vi "LLTF_Contrast_Demo_Advanced.vi"() -> ()   [LabVIEW 2017]
uses:
  PE_Filter_SDK/PE_Filter_SDK.lvlib
panel:
  out "Grating Name":string
  in  "Grating":i32=4 min=0 max=2 step=1
  in  "Wavelength":dbl=600.0 min=500.0 max=600.0 format="%.2f"
  out "Min Ext. Wavelength":dbl
  out "Max Ext. Wavelength":dbl
  in  "Move Filter":bool
  in  "Stop":bool
  out "Grating Count":i32
  out "Current System":string
  in  "Configuration File":path
  # "Filter Selection"
  # "Filter Information"
  # "Filter Control"
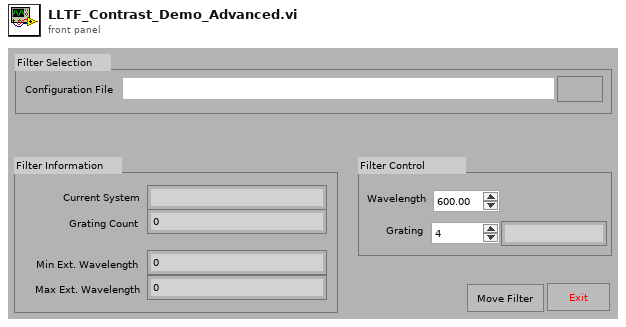
[diagram p1: front panel]
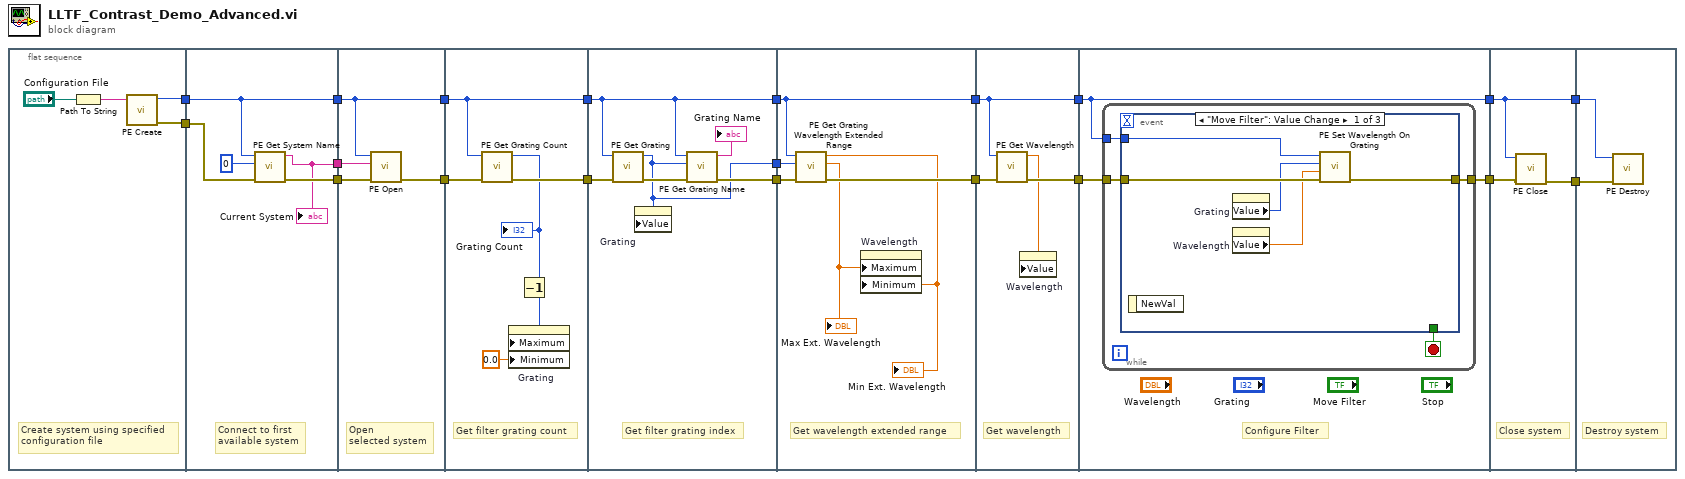
[diagram p0: block diagram]
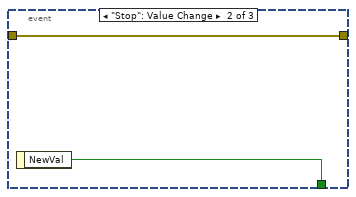
[diagram p2: hidden frame]
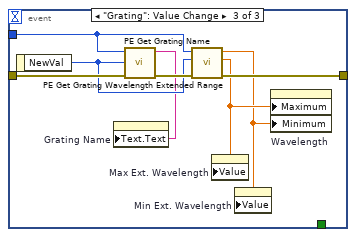
[diagram p3: hidden frame]
diagram:
  n1 = flat-sequence {
    tunnel: [w21] -> w20
    tunnel: [w22] -> w19
    tunnel: w20 -> [w29]
    tunnel: [w27] -> w17
    tunnel: [w28] -> w18
    tunnel: w19 -> [w26]
    tunnel: [w26] -> w16
    tunnel: w18 -> [w33]
    tunnel: [w30] -> w15
    tunnel: w17 -> [w32]
    tunnel: w16 -> [w31]
    tunnel: [w31] -> w14
    tunnel: w15 -> [w37]
    tunnel: [w38] -> w9
    tunnel: w14 -> [w39]
    tunnel: [w39] -> w8
    tunnel: w9 -> [w45]
    tunnel: [w43] -> w7
    tunnel: w8 -> [w42]
    tunnel: [w42] -> w6
    tunnel: [w40] -> w5
    tunnel: w7 -> [w51]
    tunnel: [w50] -> w4
    tunnel: w6 -> [w49]
    tunnel: [w49] -> w2
    tunnel: w5 -> [w48]
    tunnel: w4 -> [w54]
    tunnel: [w53] -> w3
    tunnel: w2 -> [w55]
    tunnel: [w55] -> w1
    tunnel: w3 -> [w58]
    tunnel: w1 -> [w56]
    tunnel: [w57] -> w13
    tunnel: [w56] -> w12
    tunnel: [w80] -> w11
    tunnel: w13 -> [w79]
    tunnel: w12 -> [w78]
    tunnel: [w78] -> w10
    tunnel: w11 -> [w82]
    tunnel: w10 -> [w81]
    frame #0 {
      # "Create system using specified\nconfiguration file"
      n2 = Path To String(path="Configuration File") -> (string=w23:string)
      n3 = call "PE Create.vi"("conffile"=w23) -> ("error out"=w21:errorcluster, "peHandle"=w22:u32)  [unwired: 9 in]
    }
    frame #1 {
      # "Connect to first\navailable system"
      n4 = call "PE Get System Name.vi"("error in (no error)"=w29, "index"=0, "peHandle"=w26) -> ("error out"=w28:errorcluster, "name"=w27:string)  [unwired: 6 in, 1 out]
      "Current System" <- w27
    }
    frame #2 {
      # "Open\nselected system"
      n5 = call "PE Open.vi"("error in (no error)"=w33, "name"=w32, "peHandle"=w31) -> ("error out"=w30:errorcluster)  [unwired: 8 in]
    }
    frame #3 {
      # "Get filter grating count"
      n6 = call "PE Get Grating Count.vi"("error in (no error)"=w37, "peHandle"=w39) -> ("error out"=w38:errorcluster, "count"=w35:i32)  [unwired: 8 in]
      "Grating Count" <- w35
      n7 = Decrement(x=w35) -> (x-1=w34:i32)
      n8 = property on="Grating" class="DigNum (strict)"("Maximum"=w34, "Minimum"=0.0 ("Data Entry Limits:Minimum")) -> ()  [unwired: 2 in, 2 out]
    }
    frame #4 {
      # "Get filter grating index"
      n9 = call "PE Get Grating.vi"("error in (no error)"=w45, "peHandle"=w42) -> ("error out"=w44:errorcluster, "gratingIndex"=w40:i32)  [unwired: 8 in]
      n10 = property on="Grating" class="DigNum (strict)"("Value"=w40) -> ()  [unwired: 2 in, 2 out]
      n11 = call "PE Get Grating Name.vi"("error in (no error)"=w44, "gratingIndex"=w40, "peHandle"=w42) -> ("error out"=w43:errorcluster, "name"=→"Grating Name":string)  [unwired: 7 in]
    }
    frame #5 {
      # "Get wavelength extended range"
      n12 = call "PE Get Grating Wavelength Extended Range.vi"("error in (no error)"=w51, "gratingIndex"=w48, "peHandle"=w49) -> ("error out"=w50:errorcluster, "extMaximum"=w47:dbl, "extMinimum"=w46:dbl)  [unwired: 6 in]
      "Max Ext. Wavelength" <- w47
      "Min Ext. Wavelength" <- w46
      n13 = property on="Wavelength" class="DigNum (strict)"("Maximum"=w47, "Minimum"=w46) -> ()  [unwired: 2 in, 2 out]
    }
    frame #6 {
      # "Get wavelength"
      n14 = call "PE Get Wavelength.vi"("error in (no error)"=w54, "peHandle"=w55) -> ("error out"=w53:errorcluster, "wavelength"=w52:dbl)  [unwired: 8 in]
      n15 = property on="Wavelength" class="DigNum (strict)"("Value"=w52) -> ()  [unwired: 2 in, 2 out]
    }
    frame #7 {
      # "Configure Filter"
      n16 = while {
        tunnel: w58 -> [w61]
        tunnel: [w60] -> w57
        tunnel: w56 -> [w59]
        stop <- w62 stop-if-true
        n17 = event shown="[0] \"Move Filter\": Value Change" {
          selector: _ -> [_ _ _]
          dyn-events: _ -> [_ _ _]
          timeout: _ -> [_ _ _]
          tunnel: [_ w69 _] -> w62
          tunnel: w61 -> [w66 w68 w74]
          tunnel: [w67 w68 w77] -> w60
          tunnel: w59 -> [w65 _ w70]
          event "Move Filter": Value Change {
            n18 = event-data() -> ()  [unwired: 1 in, 1 out]
            n19 = property on="Grating" class="DigNum (strict)"() -> ("Value"=w64:i32)  [unwired: 2 in, 2 out]
            n20 = property on="Wavelength" class="DigNum (strict)"() -> ("Value"=w63:dbl)  [unwired: 2 in, 2 out]
            n21 = call "PE Set Wavelength On Grating.vi"("error in (no error)"=w66, "wavelength"=w63, "gratingIndex"=w64, "peHandle"=w65) -> ("error out"=w67:errorcluster)  [unwired: 7 in]
          }
          event "Stop": Value Change {
            n22 = event-data() -> ("NewVal"=w69:bool)  [unwired: 1 in]
          }
          event "Grating": Value Change {
            n23 = event-data() -> ("NewVal"=w72:i32)  [unwired: 1 in]
            n24 = call "PE Get Grating Name.vi"("error in (no error)"=w74, "gratingIndex"=w72, "peHandle"=w70) -> ("error out"=w73:errorcluster, "name"=w71:string)  [unwired: 7 in]
            n25 = property on="Grating Name" class="Str"("Text.Text"=w71) -> ()  [unwired: 2 in, 2 out]
            n26 = call "PE Get Grating Wavelength Extended Range.vi"("error in (no error)"=w73, "gratingIndex"=w72, "peHandle"=w70) -> ("error out"=w77:errorcluster, "extMaximum"=w76:dbl, "extMinimum"=w75:dbl)  [unwired: 6 in]
            n27 = property on="Max Ext. Wavelength" class="DigNum (strict)"("Value"=w76) -> ()  [unwired: 2 in, 2 out]
            n28 = property on="Min Ext. Wavelength" class="DigNum (strict)"("Value"=w75) -> ()  [unwired: 2 in, 2 out]
            n29 = property on="Wavelength" class="DigNum (strict)"("Maximum"=w76, "Minimum"=w75) -> ()  [unwired: 2 in, 2 out]
          }
        }
      }
    }
    frame #8 {
      # "Close system"
      n30 = call "PE Close.vi"("error in (no error)"=w79, "peHandle"=w78) -> ("error out"=w80:errorcluster)  [unwired: 9 in]
    }
    frame #9 {
      # "Destroy system"
      n31 = call "PE Destroy.vi"("error in (no error)"=w82, "peHandle"=w81) -> ()  [unwired: 9 in, 1 out]
    }
  }
